vi "PointData.vi"(0 "a":dbl, 1 "e":dbl, 2 "Period":dbl, 3 "time in days":i32, 4 "Initial fi":dbl) -> (5 "Cluster XY":cluster{dbl[], dbl[]})   [LabVIEW 2020]
doc: "Returns cluster with object's position by given average distance unit (a), eccentricity (e), period, initial fi in function of time."
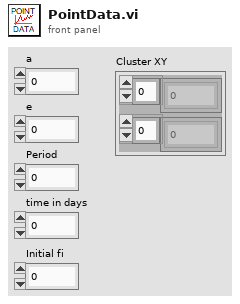
[diagram p1: front panel]
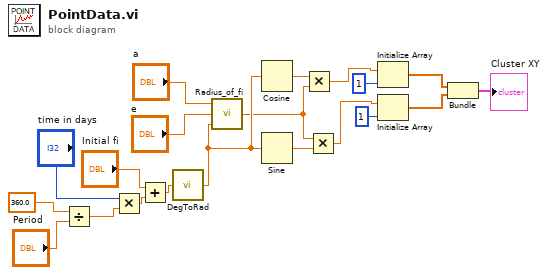
[diagram p0: block diagram]
diagram:
  n1 = Divide(x=360.0, y="Period") -> (x/y=w6:dbl)
  n2 = Multiply(x="time in days", y=w6) -> (x*y=w2:dbl)
  n3 = Add(x="Initial fi", y=w2) -> (x+y=w3:dbl)
  n4 = call "DegToRad.vi"("fi in degrees"=w3) -> ("fi in radians"=w18:dbl)
  n5 = call "Radius_of_fi.vi"("fi"=w18, "e"="e", "a"="a") -> ("r"=w17:dbl)
  n6 = Cosine(x=w18) -> (cos(x)=w16:dbl)
  n7 = Sine(x=w18) -> (sin(x)=w15:dbl)
  n8 = Multiply(x=w16, y=w17) -> (x*y=w20:dbl)
  n9 = Multiply(x=w17, y=w15) -> (x*y=w19:dbl)
  n10 = Initialize Array(w20, 1 ("dimension size")) -> (w13:dbl[])
  n11 = Initialize Array(w19, 1 ("dimension size")) -> (w14:dbl[])
  n12 = Bundle(w13, w14) -> (→"Cluster XY":cluster{dbl[], dbl[]})  [unwired: 1 in]
